vi "Find State By Name.vi"(8 "error in (no error)":errorcluster, 10 "Name":string, 11 "Tosca in":refnum<class "Parameters.lvclass">) -> (0 "error out":errorcluster, 1 "Index":i32, 2 "State":refnum<class "State.lvclass">, 3 "Tosca out":refnum<class "Parameters.lvclass">)   [LabVIEW 2015, in "Parameters.lvclass"]
uses:
  Parameters.lvclass
  State/State.lvclass
  Parameters.lvclass/Parameters.ctl
  State/State.lvclass/State.ctl
  State/Read Name.vi
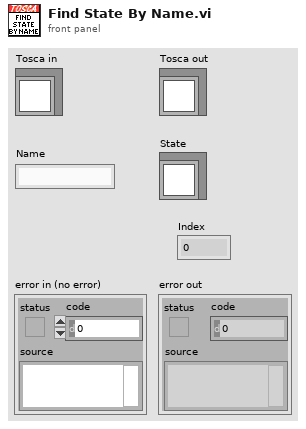
[diagram p1: front panel]
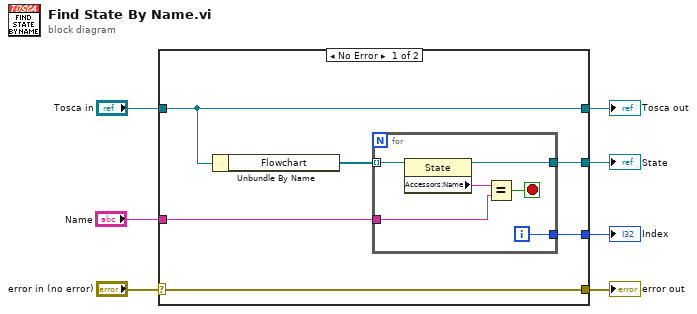
[diagram p0: block diagram]
diagram:
  n1 = case shown="No Error" "error in (no error)" {
    selector: "error in (no error)" -> [w13 w21]
    tunnel: [w13 w21] -> w6
    tunnel: [w12 w20] -> w4
    tunnel: "Tosca in" -> [w12 w20]
    tunnel: "Name" -> [w10 _]
    tunnel: [w9 _] -> w2
    tunnel: [w8 _] -> w1
    frame No Error {
      n2 = Unbundle By Name(w12) -> ("Flowchart"=w11:refnum<class "State.lvclass">[])
      n3 = for {
        tunnel: w11 -> [w19] mode=indexing
        tunnel: [w17] -> w8
        tunnel: w10 -> [w16]
        tunnel: [w15] -> w9
        i -> [w15]
        stop <- w14 stop-if-true
        n4 = property class="State"(reference=w19) -> (reference out=w17:refnum<class "State.lvclass">, "Accessors:Name"=w18:string)  [unwired: 1 in, 1 out]
        n5 = Equal?(x=w18, y=w16) -> (x = y?=w14:bool)
      }
    }
    frame Error {
    }
  }
  "error out" <- w6
  "Tosca out" <- w4
  "State" <- w1
  "Index" <- w2
